vi "Write ID.vi"(8 "error in (no error)":errorcluster, 10 "ID":string, 11 "Update Humidifier Control MSG in":refnum<class "Update Humidifier Control MSG.lvclass">) -> (0 "error out":errorcluster, 3 "Update Humidifier Control MSG out":refnum<class "Update Humidifier Control MSG.lvclass">)   [LabVIEW 2014, in "Controller.lvlib" / "Update Humidifier Control MSG.lvclass"]
uses:
  Update Humidifier Control MSG.lvclass
  Update Humidifier Control MSG.lvclass/Update Humidifier Control MSG.ctl
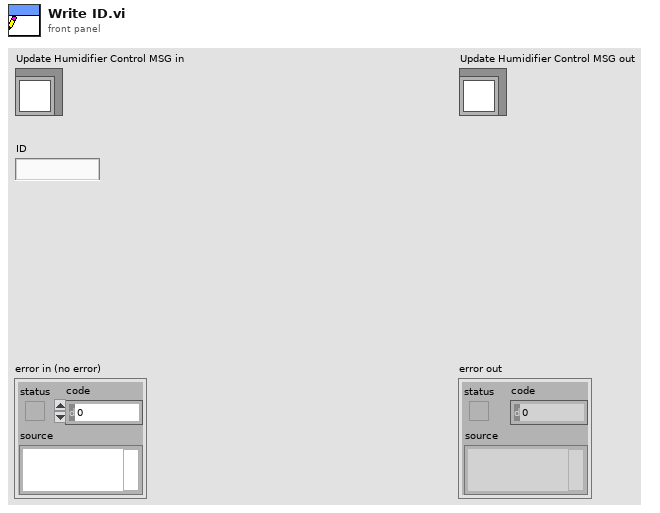
[diagram p1: front panel]
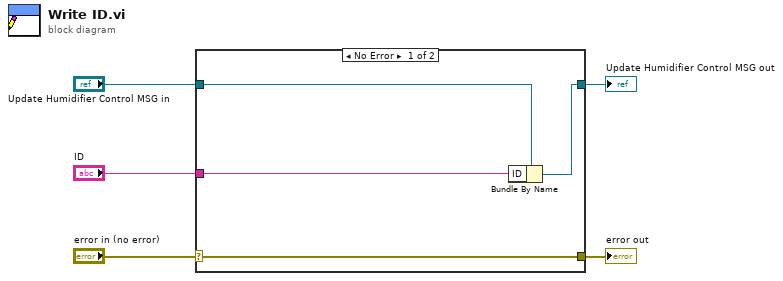
[diagram p0: block diagram]
diagram:
  n1 = case shown="No Error" "error in (no error)" {
    selector: "error in (no error)" -> [w9 w10]
    tunnel: [w9 w10] -> w4
    tunnel: [w7 w11] -> w2
    tunnel: "Update Humidifier Control MSG in" -> [w8 w11]
    tunnel: "ID" -> [w6 _]
    frame No Error {
      n2 = Bundle By Name(cluster=w8, "ID"=w6) -> (w7:refnum<class "Update Humidifier Control MSG.lvclass">)
    }
    frame Error {
    }
  }
  "error out" <- w4
  "Update Humidifier Control MSG out" <- w2
